vi "层叠顺序结构计时.vi"() -> ()   [LabVIEW 2010]
panel:
  out "当前累积数":dbl format="%.2f"
  out "循环次数":i32
  out "消耗时间":u32
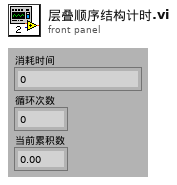
[diagram p1: front panel]
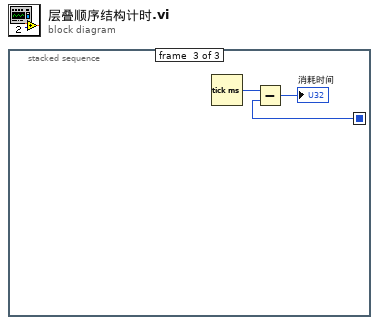
[diagram p0: block diagram]
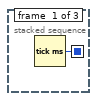
[diagram p2: hidden frame]
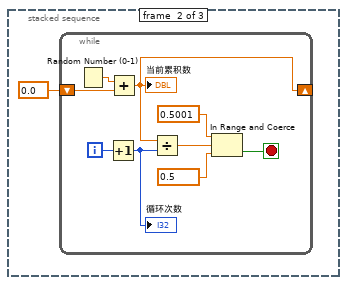
[diagram p3: hidden frame]
diagram:
  n1 = stacked-sequence {
    seq-local: [w1 _ _] -> [_ _ w13]
    frame #0 {
      n2 = Tick Count (ms)() -> (millisecond timer value=w1:u32)
    }
    frame #1 {
      n3 = while {
        shift-right: [w9] -> _
        shift-left: 0.0 -> [w10]
        i -> [w4]
        stop <- w5 stop-if-true
        n4 = Random Number (0-1)() -> (number: 0 to 1=w11:dbl)
        n5 = Increment(x=w4) -> (x+1=w3:i32)
        "循环次数" <- w3
        n6 = Add(x=w11, y=w10) -> (x+y=w9:dbl)
        "当前累积数" <- w9
        n7 = Divide(x=w9, y=w3) -> (x/y=w8:dbl)
        n8 = In Range and Coerce(upper limit=0.5001, x=w8, lower limit=0.5) -> (In Range?=w5:bool)  [unwired: 1 out]
      }
    }
    frame #2 {
      n9 = Tick Count (ms)() -> (millisecond timer value=w14:u32)
      n10 = Subtract(x=w14, y=w13) -> (x-y=→"消耗时间":u32)
    }
  }
